vi "test 4 cams.vi"() -> ()   [LabVIEW 2009]
uses:
  <vilib>/userDefined/High Color/IMAQdx.ctl
  IMAQdx Cam/IMAQdx Cam.lvclass
panel:
  in  "open settings":bool
  in  "Camera Name 4":T1="SRingPumpCamera"
  out "Image 5":T2(plugin-control)
  in  "Camera Name 3":T1="A5-Pass9 bigchip"
  out "Image 4":T2(plugin-control)
  out "Image 3":T2(plugin-control)
  in  "Camera Name 2":T1="A5-InNF"
  in  "stop":bool
  out "Image":T2(plugin-control)
  in  "Camera Name":T1="A5-InFF"
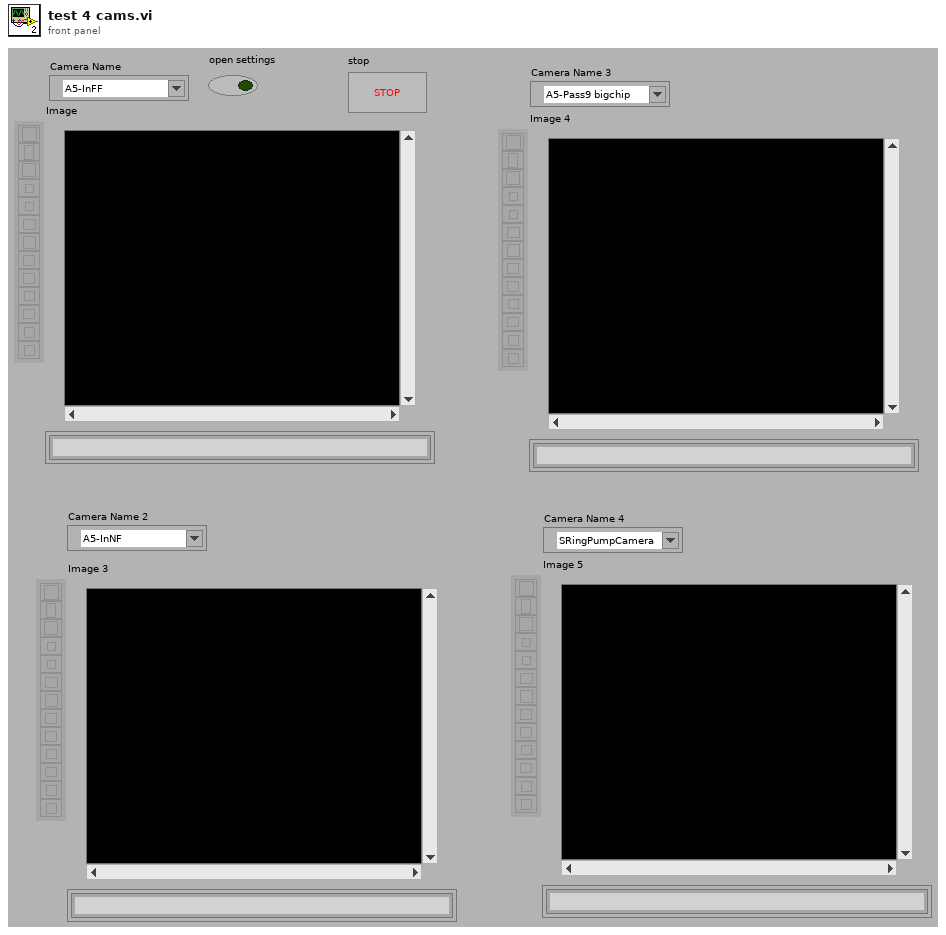
[diagram p1: front panel]
types:
  T1 = typedef "IMAQdx.ctl" = refnum<k21>
  T2 = typedef "IMAQ Image.ctl" = refnum<image>
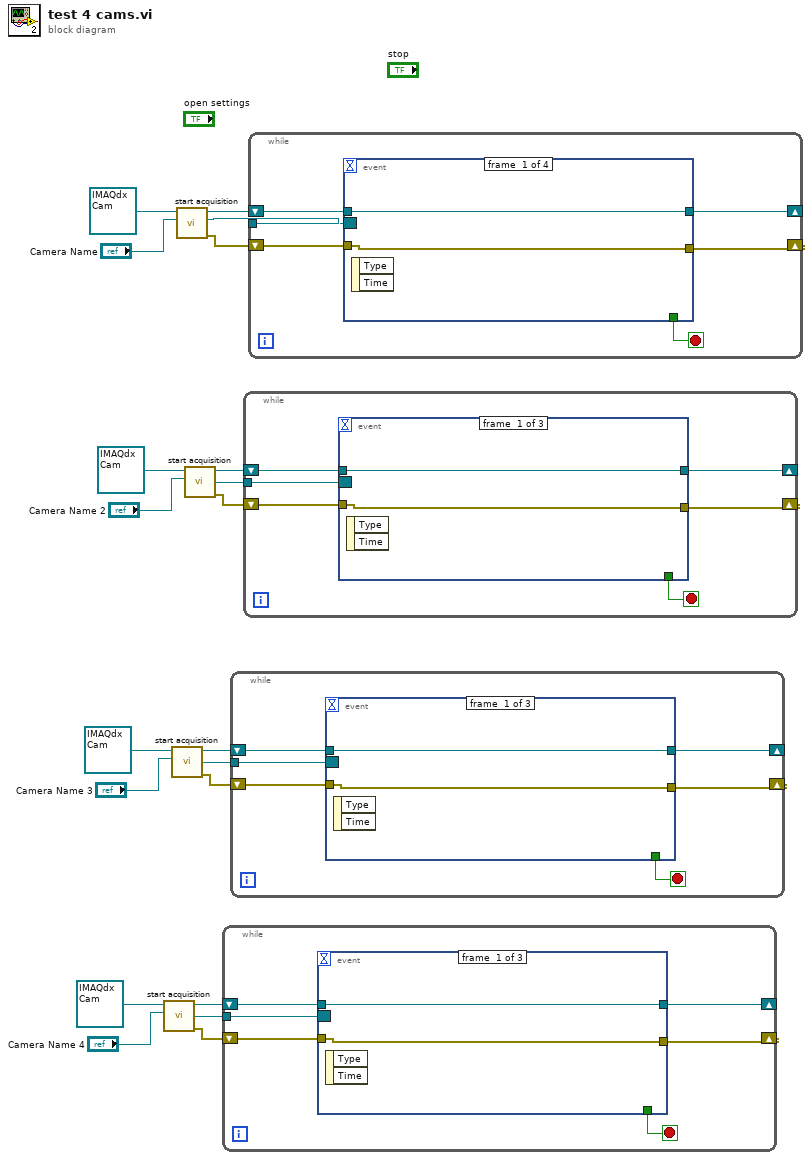
[diagram p0: block diagram]
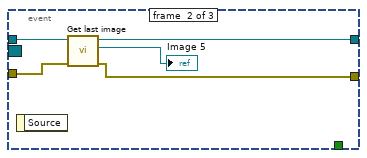
[diagram p2: hidden frame]
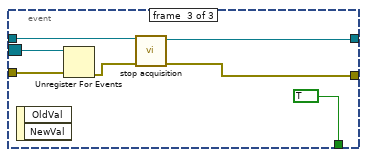
[diagram p3: hidden frame]
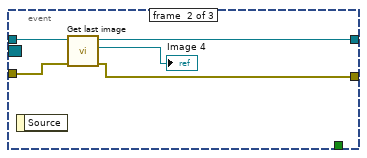
[diagram p4: hidden frame]
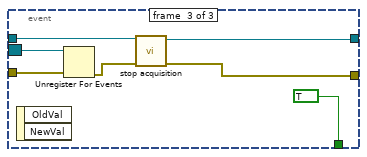
[diagram p5: hidden frame]
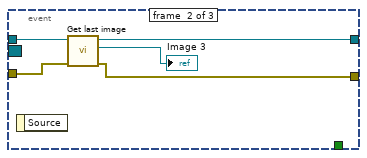
[diagram p6: hidden frame]
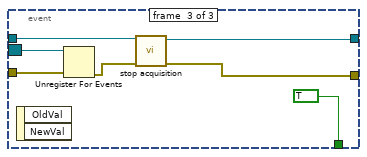
[diagram p7: hidden frame]
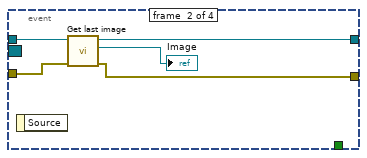
[diagram p8: hidden frame]
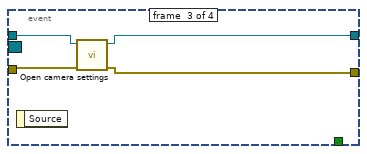
[diagram p9: hidden frame]
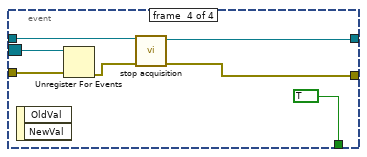
[diagram p10: hidden frame]
diagram:
  n1 = call-dynamic "start acquisition.vi"("Camera Name"="Camera Name 4", "IMAQdx Cam in"=refnum<class "IMAQdx Cam.lvclass"> refnum ("IMAQdx Cam.lvclass")) -> ("error out"=w1:errorcluster, "Event Registration Refnum"=w2:refnum<event-registration>, "IMAQdx Cam out"=w3:refnum<class "IMAQdx Cam.lvclass">)  [unwired: 7 in]
  n2 = call-dynamic "start acquisition.vi"("Camera Name"="Camera Name 3", "IMAQdx Cam in"=refnum<class "IMAQdx Cam.lvclass"> refnum ("IMAQdx Cam.lvclass")) -> ("error out"=w10:errorcluster, "Event Registration Refnum"=w9:refnum<event-registration>, "IMAQdx Cam out"=w8:refnum<class "IMAQdx Cam.lvclass">)  [unwired: 7 in]
  n3 = call-dynamic "start acquisition.vi"("Camera Name"="Camera Name", "IMAQdx Cam in"=refnum<class "IMAQdx Cam.lvclass"> refnum ("IMAQdx Cam.lvclass")) -> ("error out"=w17:errorcluster, "Event Registration Refnum"=w14:refnum<event-registration>, "IMAQdx Cam out"=w18:refnum<class "IMAQdx Cam.lvclass">)  [unwired: 7 in]
  n4 = call-dynamic "start acquisition.vi"("Camera Name"="Camera Name 2", "IMAQdx Cam in"=refnum<class "IMAQdx Cam.lvclass"> refnum ("IMAQdx Cam.lvclass")) -> ("error out"=w11:errorcluster, "Event Registration Refnum"=w12:refnum<event-registration>, "IMAQdx Cam out"=w13:refnum<class "IMAQdx Cam.lvclass">)  [unwired: 7 in]
  n5 = while {
    tunnel: w2 -> [w21]
    shift-right: [w24] -> _
    shift-left: w3 -> [w26]
    shift-right: [w23] -> _
    shift-left: w1 -> [w25]
    stop <- w22 stop-if-true
    n6 = event shown="[1] <Session Out>: FrameDone" {
      selector: w21 -> [_ _ w39]
      dyn-events: _ -> [_ _ _]
      timeout: _ -> [_ _ _]
      tunnel: w26 -> [w27 w33 w37]
      tunnel: w25 -> [w28 w32 w38]
      tunnel: [w27 w30 w35] -> w24
      tunnel: [w28 w29 w34] -> w23
      tunnel: [_ _ TRUE] -> w22
      event #0 {
        n7 = event-data() -> ()  [unwired: 1 in, 2 out]
      }
      event #1 {
        n8 = event-data() -> ()  [unwired: 1 in, 1 out]
        n9 = call-dynamic "Get last image.vi"("error in (no error)"=w32, "IMAQdx Cam in"=w33) -> ("error out"=w29:errorcluster, "Image Out"=→"Image 5":T2, "IMAQdx Cam out"=w30:refnum<class "IMAQdx Cam.lvclass">)  [unwired: 7 in]
      }
      event #2 {
        n10 = event-data() -> ()  [unwired: 1 in, 2 out]
        n11 = Unregister For Events(event registration refnum=w39, error in=w38) -> (error out=w36:errorcluster)
        n12 = call-dynamic "stop acquisition.vi"("error in (no error)"=w36, "IMAQdx Cam in"=w37) -> ("error out"=w34:errorcluster, "IMAQdx Cam out"=w35:refnum<class "IMAQdx Cam.lvclass">)  [unwired: 8 in]
      }
    }
  }
  n13 = while {
    tunnel: w9 -> [w41]
    shift-right: [w44] -> _
    shift-left: w8 -> [w46]
    shift-right: [w43] -> _
    shift-left: w10 -> [w45]
    stop <- w42 stop-if-true
    n14 = event shown="[1] <Session Out>: FrameDone" {
      selector: w41 -> [_ _ w59]
      dyn-events: _ -> [_ _ _]
      timeout: _ -> [_ _ _]
      tunnel: w46 -> [w47 w53 w57]
      tunnel: w45 -> [w48 w52 w58]
      tunnel: [w47 w50 w55] -> w44
      tunnel: [w48 w49 w54] -> w43
      tunnel: [_ _ TRUE] -> w42
      event #0 {
        n15 = event-data() -> ()  [unwired: 1 in, 2 out]
      }
      event #1 {
        n16 = event-data() -> ()  [unwired: 1 in, 1 out]
        n17 = call-dynamic "Get last image.vi"("error in (no error)"=w52, "IMAQdx Cam in"=w53) -> ("error out"=w49:errorcluster, "Image Out"=→"Image 4":T2, "IMAQdx Cam out"=w50:refnum<class "IMAQdx Cam.lvclass">)  [unwired: 7 in]
      }
      event #2 {
        n18 = event-data() -> ()  [unwired: 1 in, 2 out]
        n19 = Unregister For Events(event registration refnum=w59, error in=w58) -> (error out=w56:errorcluster)
        n20 = call-dynamic "stop acquisition.vi"("error in (no error)"=w56, "IMAQdx Cam in"=w57) -> ("error out"=w54:errorcluster, "IMAQdx Cam out"=w55:refnum<class "IMAQdx Cam.lvclass">)  [unwired: 8 in]
      }
    }
  }
  n21 = while {
    tunnel: w12 -> [w61]
    shift-right: [w64] -> _
    shift-left: w13 -> [w66]
    shift-right: [w63] -> _
    shift-left: w11 -> [w65]
    stop <- w62 stop-if-true
    n22 = event shown="[1] <Session Out>: FrameDone" {
      selector: w61 -> [_ _ w79]
      dyn-events: _ -> [_ _ _]
      timeout: _ -> [_ _ _]
      tunnel: w66 -> [w67 w73 w77]
      tunnel: w65 -> [w68 w72 w78]
      tunnel: [w67 w70 w75] -> w64
      tunnel: [w68 w69 w74] -> w63
      tunnel: [_ _ TRUE] -> w62
      event #0 {
        n23 = event-data() -> ()  [unwired: 1 in, 2 out]
      }
      event #1 {
        n24 = event-data() -> ()  [unwired: 1 in, 1 out]
        n25 = call-dynamic "Get last image.vi"("error in (no error)"=w72, "IMAQdx Cam in"=w73) -> ("error out"=w69:errorcluster, "Image Out"=→"Image 3":T2, "IMAQdx Cam out"=w70:refnum<class "IMAQdx Cam.lvclass">)  [unwired: 7 in]
      }
      event #2 {
        n26 = event-data() -> ()  [unwired: 1 in, 2 out]
        n27 = Unregister For Events(event registration refnum=w79, error in=w78) -> (error out=w76:errorcluster)
        n28 = call-dynamic "stop acquisition.vi"("error in (no error)"=w76, "IMAQdx Cam in"=w77) -> ("error out"=w74:errorcluster, "IMAQdx Cam out"=w75:refnum<class "IMAQdx Cam.lvclass">)  [unwired: 8 in]
      }
    }
  }
  n29 = while {
    tunnel: w14 -> [w81]
    shift-right: [w84] -> _
    shift-left: w18 -> [w86]
    shift-right: [w83] -> _
    shift-left: w17 -> [w85]
    stop <- w82 stop-if-true
    n30 = event shown="[2] \"open settings\": Mouse Down" {
      selector: w81 -> [_ _ _ w103]
      dyn-events: _ -> [_ _ _ _]
      timeout: _ -> [_ _ _ _]
      tunnel: w86 -> [w87 w93 w97 w101]
      tunnel: w85 -> [w88 w92 w96 w102]
      tunnel: [w87 w90 w94 w99] -> w84
      tunnel: [w88 w89 w95 w98] -> w83
      tunnel: [_ _ _ TRUE] -> w82
      event #0 {
        n31 = event-data() -> ()  [unwired: 1 in, 2 out]
      }
      event #1 {
        n32 = event-data() -> ()  [unwired: 1 in, 1 out]
        n33 = call-dynamic "Get last image.vi"("error in (no error)"=w92, "IMAQdx Cam in"=w93) -> ("error out"=w89:errorcluster, "Image Out"=→"Image":T2, "IMAQdx Cam out"=w90:refnum<class "IMAQdx Cam.lvclass">)  [unwired: 7 in]
      }
      event #2 {
        n34 = event-data() -> ()  [unwired: 1 in, 1 out]
        n35 = call-dynamic "Open camera settings.vi"("error in (no error)"=w96, "IMAQdx Cam in"=w97) -> ("error out"=w95:errorcluster, "IMAQdx Cam out"=w94:refnum<class "IMAQdx Cam.lvclass">)  [unwired: 8 in]
      }
      event #3 {
        n36 = event-data() -> ()  [unwired: 1 in, 2 out]
        n37 = Unregister For Events(event registration refnum=w103, error in=w102) -> (error out=w100:errorcluster)
        n38 = call-dynamic "stop acquisition.vi"("error in (no error)"=w100, "IMAQdx Cam in"=w101) -> ("error out"=w98:errorcluster, "IMAQdx Cam out"=w99:refnum<class "IMAQdx Cam.lvclass">)  [unwired: 8 in]
      }
    }
  }
